vi "get_time-v02.vi"() -> (2 "time output":string, 3 "pure text output":string)   [LabVIEW 2019]
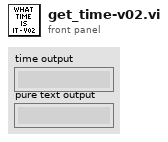
[diagram p1: front panel]
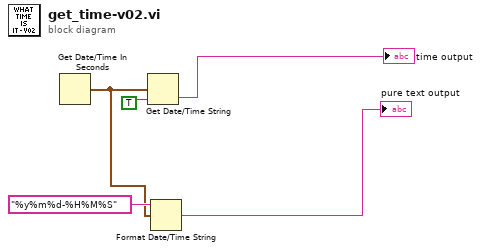
[diagram p0: block diagram]
diagram:
  n1 = Get Date/Time In Seconds() -> (seconds since 1Jan1904=w2:timestamp)
  n2 = Get Date/Time String(seconds (now)=w2, want seconds? (F)=TRUE) -> (time string=→"time output":string)  [unwired: 1 in, 1 out]
  n3 = Format Date/Time String(time format string (%c)="%y%m%d-%H%M%S", seconds (now)=w2) -> (date/time string=→"pure text output":string)  [unwired: 1 in]
